vi "Add Resistive card.vi"(8 "error in (no error)":errorcluster, 11 "Node Ptr":u64 format="%.0x") -> (0 "error out":errorcluster)   [LabVIEW 2014, in "SLSC configuration System Explorer.lvlib"]
uses:
  SLSC configuration System Explorer.lvlib
  Shared/Constants.vi
  Shared/SLSC configuration Shared.lvlib
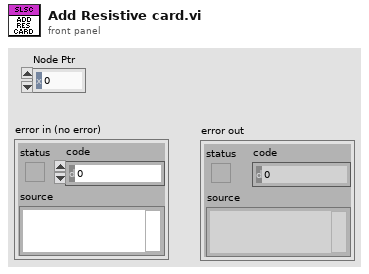
[diagram p1: front panel]
types:
  T1 = typedef "SLSC configuration Shared.lvlib/Card Position.ctl" = cluster{"Rack #":u8, "Slot #":T2}
  T2 = typedef "SLSC configuration Shared.lvlib/Slot #.ctl" = u8
  T3 = typedef "Custom Device API.lvlib/Custom Device Item Ref.ctl" = u64
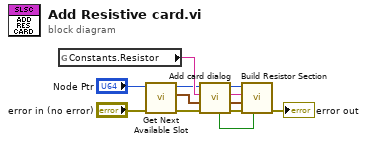
[diagram p0: block diagram]
diagram:
  n1 = global read "Constants.vi" "Constants.Resistor"() -> (w9:string)
  n2 = call "Get Next Available Slot.vi"("error in (no error)"="error in (no error)", "Device Ref in"="Node Ptr") -> ("error out"=w4:errorcluster, "Next Open Slot"=w1:T1, "Device Ref out"=w2:T3)  [unwired: 7 in]
  n3 = call "Add card dialog.vi"("error in (no error)"=w4, "Card Position"=w1, "Card Type in"=w9, "Node Ptr"=w2) -> ("error out"=w12:errorcluster, "Card Position out"=w7:T1, "Name out"=w8:string, "Node Ptr out"=w11:u64, "Cancelled?"=w6:bool)  [unwired: 3 in]
  n4 = call "Build Resistor Section.vi"("Cancelled?"=w6, "error in (no error)"=w12, "Card Position"=w7, "Name"=w8, "Node Ptr"=w11) -> ("error out"=→"error out":errorcluster)  [unwired: 6 in]
